vi "Configure Session.vi"(8 "error in":errorcluster, 11 "Plugin in":refnum<class "FFT.lvclass">) -> (0 "error out":errorcluster, 3 "Plugin out":refnum<class "FFT.lvclass">)   [LabVIEW 2024, in "FFT.lvlib" / "FFT.lvclass"]
uses:
  FFT.lvclass
  FFT Buffer Manager Function.ctl
  FFT.lvclass/FFT.ctl
  <vilib>/FlexLogger/SDK/PluginSDK.lvlibp/PEFClasses/SDK/Channel/Data Type_v2.ctl
  <vilib>/FlexLogger/SDK/PluginSDK.lvlibp/PEFClasses/SDK/Consumer Channel/Consumer Channel.lvclass
  C:/Program Files/National Instruments/LabVIEW 2024/vi.lib/FlexLogger/SDK/PluginSDK.lvlibp/PEFClasses/SDK/Channel/Channel.lvclass
  <vilib>/FlexLogger/SDK/PluginSDK.lvlibp/PEFClasses/SDK/Producer Channel/Producer Channel.lvclass
  <vilib>/FlexLogger/SDK/PluginSDK.lvlibp/PEFClasses/SDK/Channel/Read Public Parameters.vi
  FFT Globals.vi
  <vilib>/FlexLogger/SDK/PluginSDK.lvlibp/PEFClasses/SDK/Producer Channel/Create Producer Channel_v2.vi
  <vilib>/FlexLogger/SDK/PluginSDK.lvlibp/PEFClasses/SDK/Channel/ParameterAccess/Write Boolean.vi
  <vilib>/FlexLogger/SDK/PluginSDK.lvlibp/PEFClasses/SDK/Channel/ParameterAccess/Write I32.vi
  <vilib>/FlexLogger/SDK/PluginSDK.lvlibp/PEFClasses/SDK/Parameters/Parameters.lvclass
  <vilib>/FlexLogger/SDK/PluginSDK.lvlibp
  <vilib>/FlexLogger/SDK/PluginSDK.lvlibp/PEFClasses/SDK/Plugin/Plugin.lvclass
  <vilib>/FlexLogger/SDK/PluginSDK.lvlibp/PEFClasses/SDK/Channel/Channel.lvclass
  C:/Program Files/National Instruments/LabVIEW 2024/vi.lib/FlexLogger/SDK/PluginSDK.lvlibp/PEFClasses/SDK/Plugin/Plugin.lvclass
  C:/Program Files/National Instruments/LabVIEW 2024/vi.lib/FlexLogger/SDK/PluginSDK.lvlibp/PEFClasses/SDK/Producer Channel/Producer Channel.lvclass
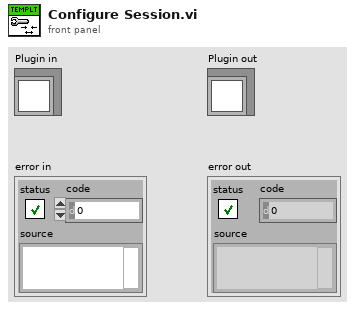
[diagram p1: front panel]
types:
  T1 = typedef "FFT.lvlib/FFT.lvclass/FFT Buffer Manager Function.ctl" = enum16{"Get Data", "Buffer Data", "Reset Data"}
  T2 = typedef "PluginSDK.lvlibp/Channel.lvclass/Data Type_v2.ctl" = u16
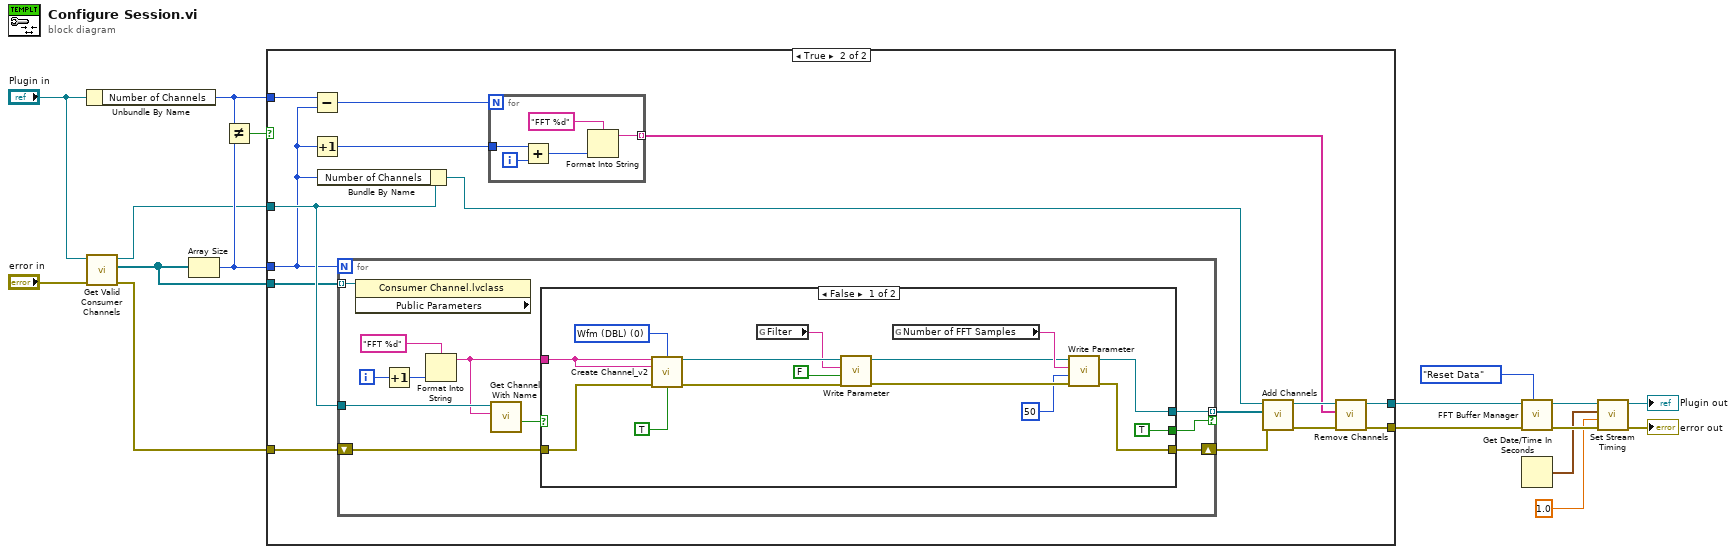
[diagram p0: block diagram]
diagram:
  n1 = Unbundle By Name("Plugin in") -> ("Number of Channels"=w14:i32)
  n2 = call <vilib>:"Get Valid Consumer Channels.vi"("error in (no error)"="error in", "Plugin in"="Plugin in") -> ("error out"=w4:errorcluster, "Channels"=w1:refnum<class "Consumer Channel.lvclass">[], "Plugin out"=w5:refnum<class "FFT.lvclass">)  [unwired: 7 in]
  n3 = Array Size(array=w1) -> (size(s)=w12:i32)
  n4 = Not Equal?(x=w14, y=w12) -> (x != y?=w16:bool)
  n5 = case shown="True" w16 {
    tunnel: [w18 w23] -> w15
    tunnel: [w19 w22] -> w13
    tunnel: w14 -> [_ w32]
    tunnel: w5 -> [w19 w29]
    tunnel: w12 -> [_ w28]
    tunnel: w4 -> [w18 w21]
    tunnel: w1 -> [_ w20]
    frame False {
    }
    frame True {
      n6 = Subtract(x=w32, y=w28) -> (x-y=w31:i32)
      n7 = Increment(x=w28) -> (x+1=w30:i32)
      n8 = Bundle By Name(cluster=w29, "Number of Channels"=w28) -> (w27:refnum<class "FFT.lvclass">)
      n9 = for {
        N: w28 -> [_]
        tunnel: [w50] -> w34 mode=indexing if=w41
        shift-right: [w49] -> w33
        shift-left: w21 -> [w47]
        tunnel: w29 -> [w44]
        tunnel: w20 -> [w40] mode=indexing
        i -> [w46]
        n10 = property class="Consumer Channel.lvclass" props=["Public Parameters"](reference=w40) -> ()  [unwired: 1 in, 3 out]
        n11 = Increment(x=w46) -> (x+1=w45:i32)
        n12 = Format Into String(format string="FFT %d", w45) -> (resulting string=w43:string)  [unwired: 2 in, 1 out]
        n13 = call <vilib>:"Get Channel With Name.vi"("Name"=w43, "Plugin in"=w44) -> ("Found?"=w42:bool)  [unwired: 7 in, 2 out]
        n14 = case shown="False" w42 {
          tunnel: [w54 _] -> w50
          tunnel: [w52 w66] -> w49
          tunnel: w47 -> [w63 w66]
          tunnel: w43 -> [w62 _]
          tunnel: [TRUE _] -> w41
          frame False {
            w65 = T2 0 items=["Wfm (DBL)", "Wfm (Digital)", "String"] ("Data Type")
            n15 = call-poly <vilib>:"Create Channel_v2.vi"("Unique Channel Identifier"=w62, "Data Type"=w65, "Default Channel Name"=w62, "error in (no error)"=w63, "Can Disable?"=TRUE) -> ("Producer Channel"=w60:refnum<class "Producer Channel.lvclass">, "error out"=w59:errorcluster)  [unwired: 9 in]
            n16 = global read "FFT Globals.vi" "Filter"() -> (w58:string)
            n17 = call-poly <vilib>:"Write Parameter.vi"("error in (no error)"=w59, "Value"=FALSE, "Name"=w58, "Channel in"=w60) -> ("error out"=w53:errorcluster, "Channel out"=w55:refnum<class "Producer Channel.lvclass">)  [unwired: 6 in]
            n18 = global read "FFT Globals.vi" "Number of FFT Samples"() -> (w56:string)
            n19 = call-poly <vilib>:"Write Parameter.vi"("error in (no error)"=w53, "Value"=50, "Name"=w56, "Channel in"=w55) -> ("error out"=w52:errorcluster, "Channel out"=w54:refnum<class "Producer Channel.lvclass">)  [unwired: 6 in]
          }
          frame True {
          }
        }
      }
      n20 = for {
        N: w31 -> [_]
        tunnel: w30 -> [w38]
        tunnel: [w35] -> w25 mode=indexing
        i -> [w37]
        n21 = Add(x=w38, y=w37) -> (x+y=w36:i32)
        n22 = Format Into String(format string="FFT %d", w36) -> (resulting string=w35:string)  [unwired: 2 in, 1 out]
      }
      n23 = call <vilib>:"Add Channels.vi"("error in (no error)"=w33, "Channels"=w34, "Plugin in"=w27) -> ("error out"=w24:errorcluster, "Plugin out"=w26:refnum<class "FFT.lvclass">)  [unwired: 7 in]
      n24 = call-dynamic "Remove Channels.vi"("error in (no error)"=w24, "Unique Channel Identifiers to Delete"=w25, "Plugin in"=w26) -> ("error out"=w23:errorcluster, "Plugin out"=w22:refnum<class "FFT.lvclass">)  [unwired: 7 in]
    }
  }
  n25 = call "FFT Buffer Manager.vi"("Function"=FFT_Buffer_Manager_Function."Reset Data", "error in"=w15, "Plugin in"=w13) -> ("error out"=w9:errorcluster, "Plugin out"=w11:refnum<class "FFT.lvclass">)  [unwired: 5 in, 2 out]
  n26 = Get Date/Time In Seconds() -> (seconds since 1Jan1904=w6:timestamp)
  n27 = call-dynamic "Set Stream Timing.vi"("error in (no error)"=w9, "dt(sec)"=1.0, "Start Time"=w6, "Plugin in"=w11) -> ("error out"=→"error out":errorcluster, "Plugin out"=→"Plugin out":refnum<class "FFT.lvclass">)  [unwired: 6 in]
